vi "Manual Assembly - Copy.vi"() -> ()   [LabVIEW 2019]
uses:
  Classes/Routine/Routine Enum.ctl
  Classes/Assembly/Assembly Run.lvclass
  Classes/Workspace/Fixture Enum.ctl
  Classes/Controller/Controller.lvclass
  Classes/Workspace/Fixture.lvclass
  Classes/Routine/Routine.lvclass
panel:
  out "Array 3":string[][](array[string])
  out "Array 2":string[][](array[string])
  in  "?":bool
  in  "Update":bool
  in  "Stage":i32(listbox)=-1
  in  "Routine":T1=enum."Dispense on Plate"
  in  "Stop":bool
  in  "Remove":bool
  in  "Add":bool
  in  "Go":bool
  # "6 Inch"
  # "8 Inch"
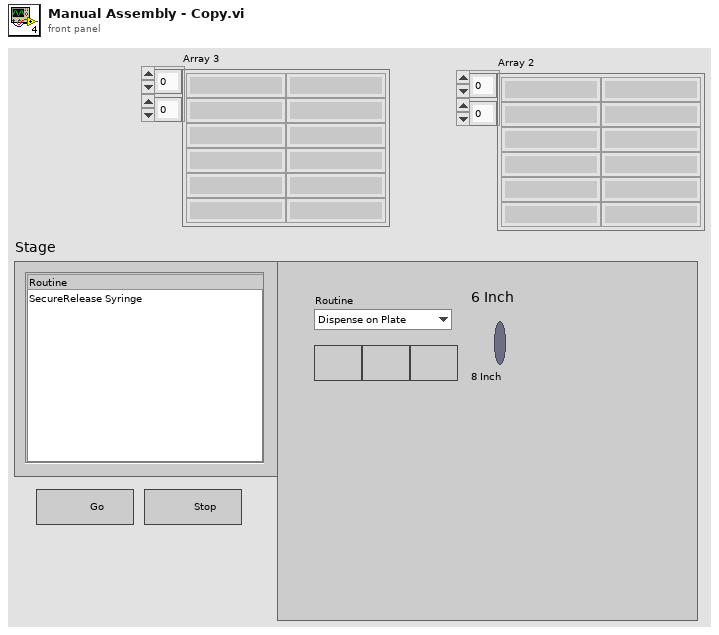
[diagram p1: front panel]
types:
  T1 = typedef "Routine.lvclass/Routine Enum.ctl" = enum16{"Primary Pick Up", "Pick Up All", "Put Down Secondary", "Put Down All", "Release Syringe", "Secondary Pick Up", "Secure Syringe", "Dispense on Plate", "Dispense on Kapton", "Dispense on Sensor", "Dispense Offset"}
  T2 = typedef "Controller.lvclass/Controllers.ctl" = cluster{"I-O.lvclass":refnum<class "I-O.lvclass">, "Dispenser.lvclass":refnum<class "Dispenser.lvclass">, "Gantry":refnum<k24>}
  T3 = typedef "Fixture.lvclass/Fixture Enum.ctl" = enum16{"Assembly Tray", "Syringe Space", "Component", "Pick Up Tool", "Current Position"}
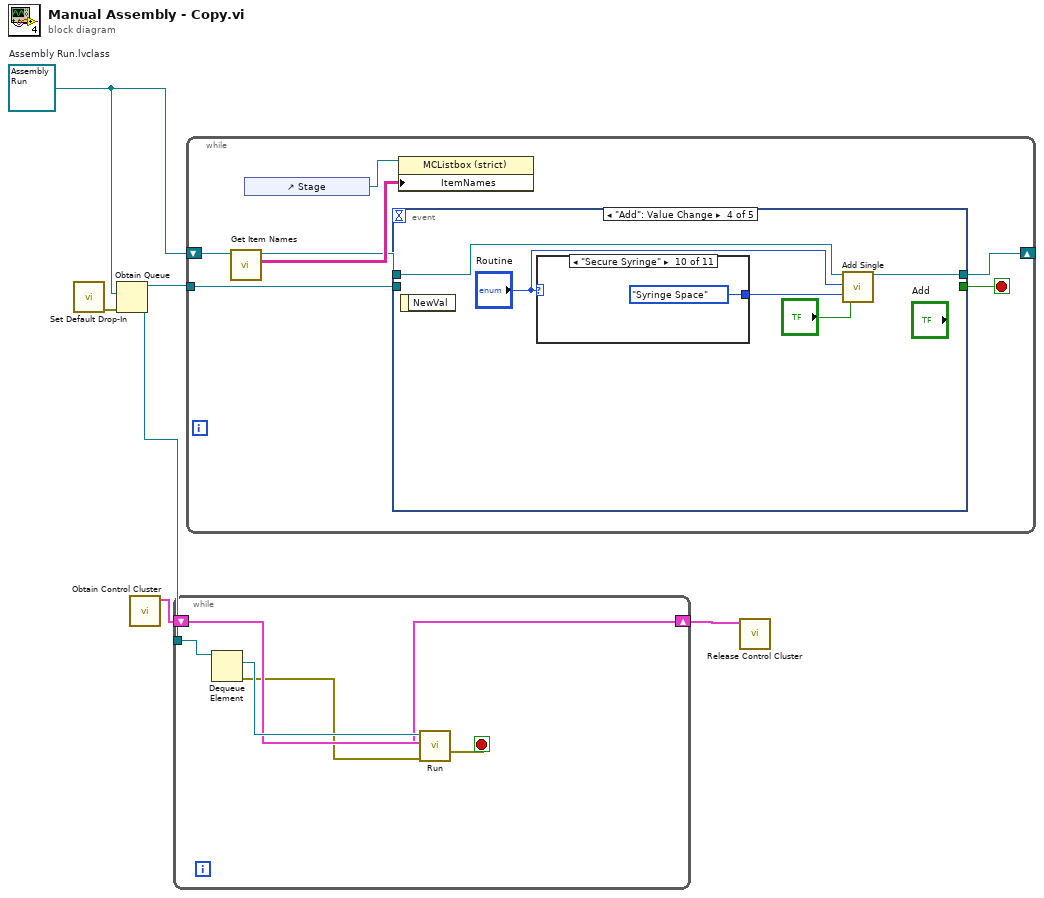
[diagram p0: block diagram]
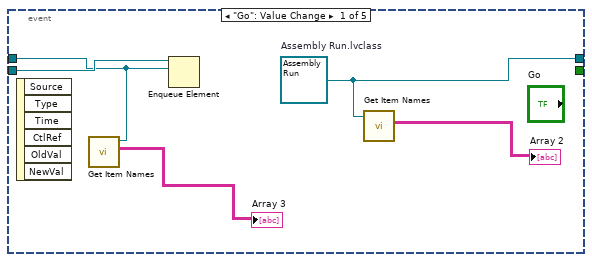
[diagram p2: hidden frame]
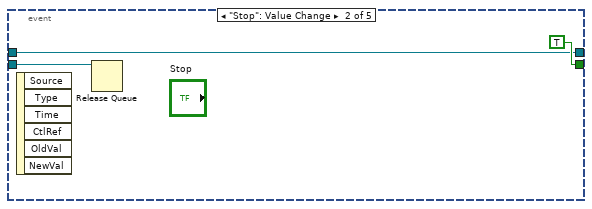
[diagram p3: hidden frame]
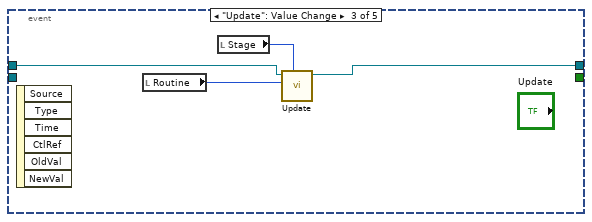
[diagram p4: hidden frame]
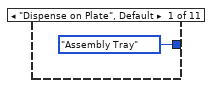
[diagram p5: hidden frame]
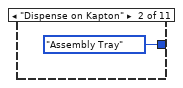
[diagram p6: hidden frame]
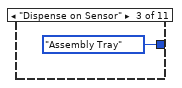
[diagram p7: hidden frame]
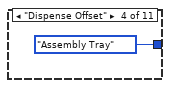
[diagram p8: hidden frame]
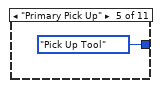
[diagram p9: hidden frame]
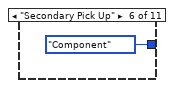
[diagram p10: hidden frame]
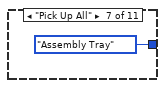
[diagram p11: hidden frame]
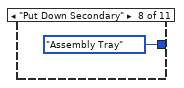
[diagram p12: hidden frame]
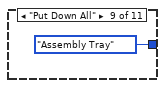
[diagram p13: hidden frame]
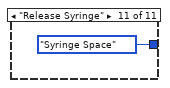
[diagram p14: hidden frame]
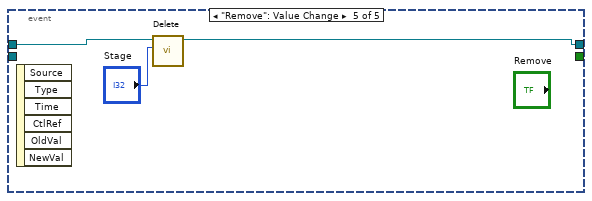
[diagram p15: hidden frame]
diagram:
  w1 = refnum<class "Assembly Run.lvclass"> refnum  # Assembly Run.lvclass
  n1 = call "Set Default Drop-In.vi"() -> ("error out"=w2:errorcluster)  [unwired: 11 in]
  n2 = Obtain Queue(element data type=w1, error in (no error)=w2) -> (queue out=w5:refnum<queue>)  [unwired: 3 in, 2 out]
  n3 = call "Obtain Control Cluster.vi"() -> ("Control Out"=w4:T2)  [unwired: 11 in]
  n4 = while {
    tunnel: w5 -> [w11]
    shift-right: [w6] -> w3
    shift-left: w4 -> [w9]
    stop <- w7 stop-if-true
    n5 = Dequeue Element(queue=w11) -> (element=w10:refnum<class "Assembly Run.lvclass">, error out=w8:errorcluster)  [unwired: 2 in, 2 out]
    n6 = call-dynamic "Run.vi"("error in (no error)"=w8, "Control In"=w9, "Assembly In"=w10) -> ("error out"=w7:errorcluster, "Control Out"=w6:T2)  [unwired: 6 in, 1 out]
  }
  n7 = while {
    shift-right: [w12] -> _
    shift-left: w1 -> [w14]
    tunnel: w5 -> [w17]
    stop <- w18 stop-if-true
    n8 = call "Get Item Names.vi"("Assembly Run in"=w14) -> ("Item names"=w16:string[][], "Assembly Run out"=w13:refnum<class "Assembly Run.lvclass">)  [unwired: 8 in, 1 out]
    n9 = control-ref of="Stage"() -> (w15:refnum<vi>)
    n10 = event shown="[3] \"Add\": Value Change" {
      selector: _ -> [_ _ _ _ _]
      dyn-events: _ -> [_ _ _ _ _]
      timeout: _ -> [_ _ _ _ _]
      tunnel: [_ TRUE _ _ _] -> w18
      tunnel: w13 -> [w20 w25 w30 w35 w49]
      tunnel: [w22 w25 w29 w34 w48] -> w12
      tunnel: w17 -> [w23 w24 _ _ _]
      event "Go": Value Change {
        w22 = refnum<class "Assembly Run.lvclass"> refnum  # Assembly Run.lvclass
        n11 = event-data() -> ()  [unwired: 1 in, 6 out]
        n12 = call "Get Item Names.vi"("Assembly Run in"=w20) -> ("Item names"=→"Array 3":string[][])  [unwired: 8 in, 2 out]
        n13 = Enqueue Element(queue=w23, element=w20) -> ()  [unwired: 2 in, 3 out]
        n14 = call "Get Item Names.vi"("Assembly Run in"=w22) -> ("Item names"=→"Array 2":string[][])  [unwired: 8 in, 2 out]
      }
      event "Stop": Value Change {
        n15 = event-data() -> ()  [unwired: 1 in, 6 out]
        n16 = Release Queue(queue=w24) -> ()  [unwired: 2 in, 3 out]
      }
      event "Update": Value Change {
        n17 = event-data() -> ()  [unwired: 1 in, 6 out]
        n18 = local read "Routine"() -> (w28:T1)
        n19 = local read "Stage"() -> (w27:i32)
        n20 = call "Update.vi"("Row"=w27, "Routine"=w28, "Assembly Run in"=w30) -> ("Assembly Run out"=w29:refnum<class "Assembly Run.lvclass">)  [unwired: 7 in, 1 out]
      }
      event "Add": Value Change {
        n21 = event-data() -> ()  [unwired: 1 in, 1 out]
        n22 = case shown="\"Secure Syringe\"" "Routine" {
          tunnel: [Fixture_Enum."Assembly Tray" ("Fixture") Fixture_Enum."Assembly Tray" ("Fixture") Fixture_Enum."Assembly Tray" ("Fixture") Fixture_Enum."Assembly Tray" ("Fixture") Fixture_Enum."Pick Up Tool" ("Fixture") Fixture_Enum."Component" ("Fixture") Fixture_Enum."Assembly Tray" ("Fixture") Fixture_Enum."Assembly Tray" ("Fixture") Fixture_Enum."Assembly Tray" ("Fixture") Fixture_Enum."Syringe Space" ("Fixture") Fixture_Enum."Syringe Space" ("Fixture")] -> w31
          frame "Dispense on Plate", Default {
          }
          frame "Dispense on Kapton" {
          }
          frame "Dispense on Sensor" {
          }
          frame "Dispense Offset" {
          }
          frame "Primary Pick Up" {
          }
          frame "Secondary Pick Up" {
          }
          frame "Pick Up All" {
          }
          frame "Put Down Secondary" {
          }
          frame "Put Down All" {
          }
          frame "Secure Syringe" {
          }
          frame "Release Syringe" {
          }
        }
        n23 = call-dynamic "Add Single.vi"("UI in"=w35, "Routine"="Routine", "Fixture"=w31, "Module Size"="?") -> ("UI out"=w34:refnum<class "Assembly Run.lvclass">)  [unwired: 14 in, 1 out]
      }
      event "Remove": Value Change {
        n24 = event-data() -> ()  [unwired: 1 in, 6 out]
        n25 = call "Delete.vi"("Index"="Stage", "Assembly In"=w49) -> ("Assembly Out"=w48:refnum<class "Assembly Run.lvclass">)  [unwired: 8 in, 1 out]
      }
    }
    n26 = property class="MCListbox (strict)"(reference=w15, "ItemNames"=w16) -> ()  [unwired: 1 in, 2 out]
  }
  n27 = call "Release Control Cluster.vi"("output cluster"=w3) -> ()  [unwired: 11 in]
